vi "administrator.vi"(0 "vi path":path) -> ()   [LabVIEW 2010]
panel:
  in  "Test Number":string
  in  "User":string
  in  "OK Button":bool
  out "File path":string
  out "User Name 2":string caption="User Name"
  in  "Exit Modify":bool
  in  "Replace":bool
  in  "New Password":string
  in  "New Name":string
  in  "New Group":u16(ring) items=["admin", "user"]
  out "Username                  Tests Completed   Priviledges":string[][](array[string])
  in  "Exit":bool
  in  "Modify":bool
  out "Password":string
  out "Group":u16(ring) items=["admin", "user"]
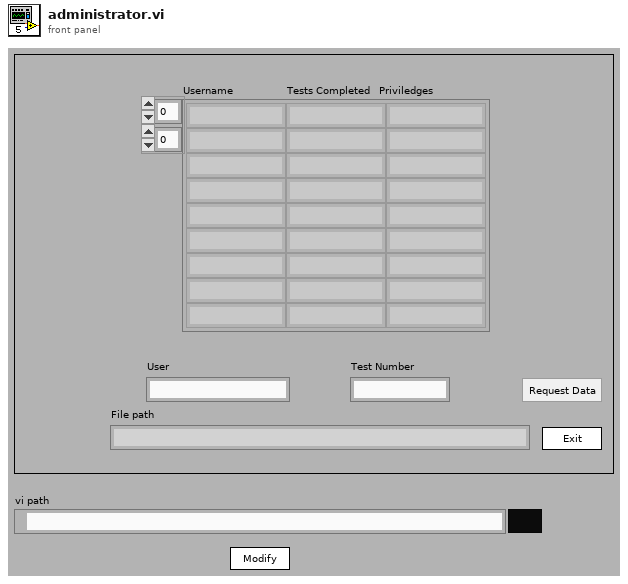
[diagram p1: front panel]
types:
  T1 = enum16{"open", "open or create", "create or replace", "create", "open (read only)"}
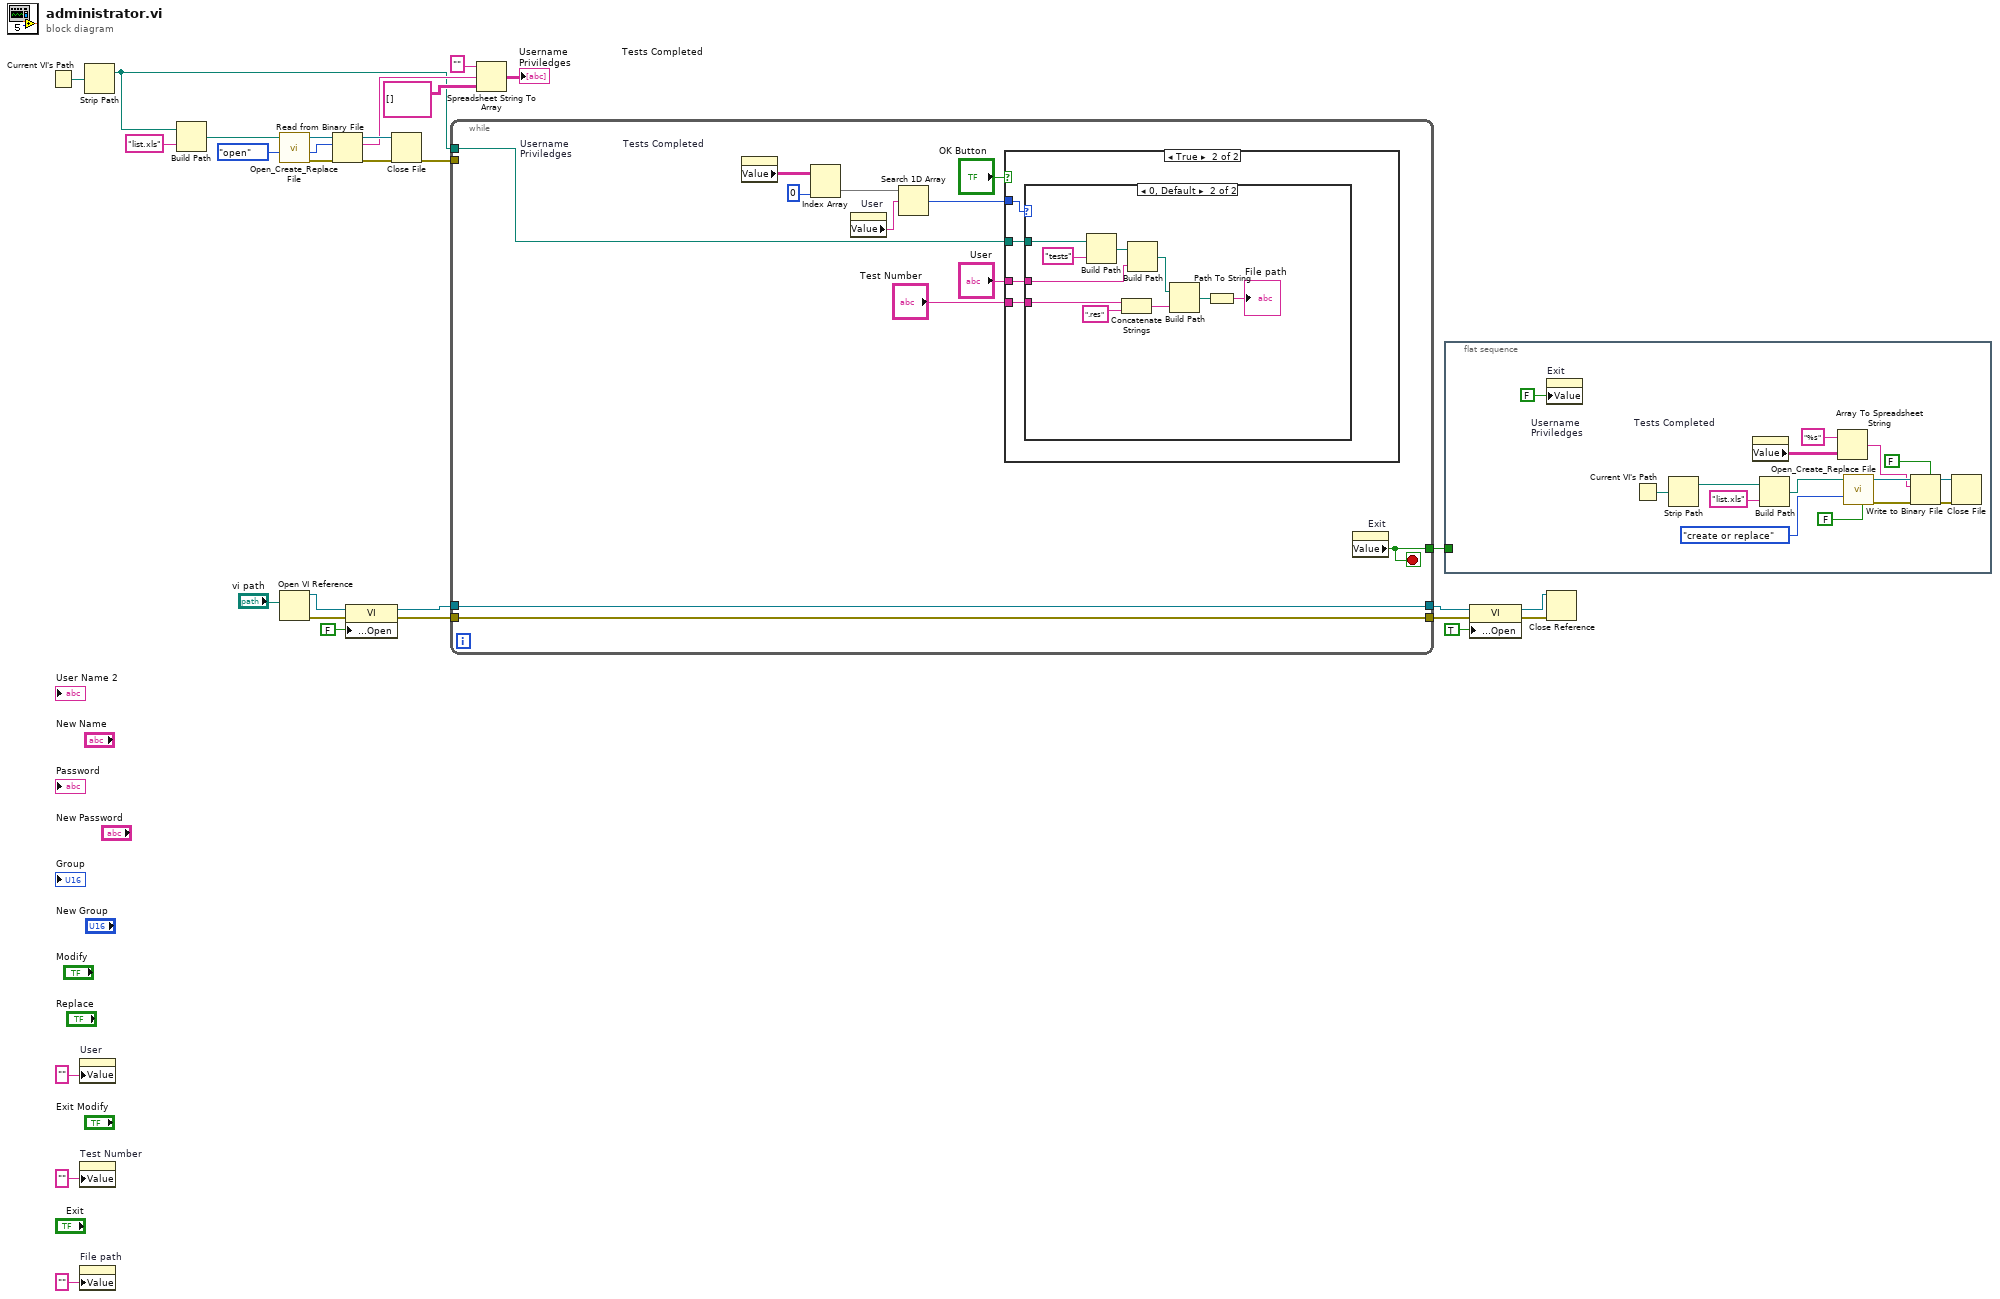
[diagram p0: block diagram]
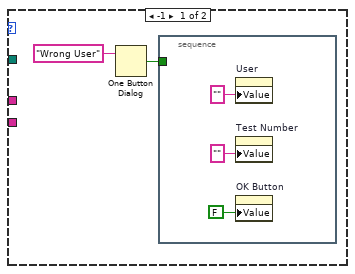
[diagram p3: hidden frame]
diagram:
  n1 = Current VI's Path() -> (path=w7:path)
  n2 = property on="User" class="Str"("Value"="" ("String")) -> ()  [unwired: 2 in, 2 out]
  n3 = property on="Test Number" class="Str"("Value"="" ("String")) -> ()  [unwired: 2 in, 2 out]
  n4 = property on="File path" class="Str"("Value"="" ("String")) -> ()  [unwired: 2 in, 2 out]
  n5 = Strip Path(path=w7) -> (stripped path=w1:path)  [unwired: 1 out]
  n6 = Build Path(base path=w1, name or relative path="list.xls") -> (appended path=w5:path)
  n7 = call <vilib>:"Open_Create_Replace File.vi"("function (open:0)"=T1."open", "file path"=w5) -> ("error out"=w30:errorcluster, "file size (bytes)"=w26:i32, "refnum"=w29:refnum<file>)  [unwired: 6 in, 1 out]
  n8 = Open VI Reference(vi path="vi path") -> (vi reference=w17:refnum<vi>, error out=w16:errorcluster)  [unwired: 5 in]
  n9 = Read from Binary File(8:w30, 10:w26, 11:w29) -> (0:w28:errorcluster, 2:w25:string, 3:w27:refnum<file>)  [unwired: 3 in, 1 out]
  n10 = property class="VI"(reference=w17, error in=w16, "Front Panel Window:Open"=FALSE) -> (reference out=w14:refnum<vi>, error out=w13:errorcluster)
  n11 = Close File(refnum=w27, error in=w28) -> (error out=w20:errorcluster)  [unwired: 1 out]
  n12 = while {
    tunnel: w20 -> [_]
    tunnel: [w42] -> w19
    tunnel: w14 -> [w41]
    tunnel: w13 -> [w40]
    tunnel: [w41] -> w11
    tunnel: [w40] -> w10
    tunnel: w1 -> [w39]
    stop <- w42 stop-if-true
    n13 = property on="Username                  Tests Completed   Priviledges" class="Arr (strict)"() -> ("Value"=w32:string[][])  [unwired: 2 in, 2 out]
    n14 = Index Array(array=w32, index (col)=0 ("disabled index (col)")) -> (element=w33:string[])  [unwired: 1 in]
    n15 = property on="User" class="Str"() -> ("Value"=w35:string)  [unwired: 2 in, 2 out]
    n16 = Search 1D Array(1D array=w33, element=w35) -> (index of element=w31:i32)  [unwired: 1 in]
    n17 = case shown="True" "OK Button" {
      tunnel: "User" -> [_ w46]
      tunnel: "Test Number" -> [_ w45]
      tunnel: w39 -> [_ w44]
      tunnel: w31 -> [_ w43]
      frame False {
      }
      frame True {
        n18 = case shown="0, Default" w43 {
          tunnel: w46 -> [_ w55]
          tunnel: w45 -> [_ w57]
          tunnel: w44 -> [_ w53]
          frame -1 {
            n19 = One Button Dialog(message="Wrong User") -> (true=w47:bool)  [unwired: 1 in]
            n20 = stacked-sequence {
              tunnel: w47 -> [_]
              frame #0 {
                n21 = property on="User" class="Str"("Value"="" ("Password")) -> ()  [unwired: 2 in, 2 out]
                n22 = property on="Test Number" class="Str"("Value"="" ("Password")) -> ()  [unwired: 2 in, 2 out]
                n23 = property on="OK Button" class="Bool"("Value"=FALSE ("true")) -> ()  [unwired: 2 in, 2 out]
              }
            }
          }
          frame 0, Default {
            n24 = Build Path(base path=w53, name or relative path="tests") -> (appended path=w54:path)
            n25 = Concatenate Strings(w57, ".res" ("string")) -> (w61:string)
            n26 = Build Path(base path=w54, name or relative path=w55) -> (appended path=w58:path)
            n27 = Build Path(base path=w58, name or relative path=w61) -> (appended path=w59:path)
            n28 = Path To String(path=w59) -> (string=→"File path":string)
          }
        }
      }
    }
    n29 = property on="Exit" class="Bool (strict)"() -> ("Value"=w42:bool)  [unwired: 2 in, 2 out]
  }
  n30 = Spreadsheet String To Array(format string="", spreadsheet string=w25, array type (2D Dbl)=string[][] []) -> (array=→"Username                  Tests Completed   Priviledges":string[][])  [unwired: 1 in]
  n31 = flat-sequence {
    tunnel: w19 -> [_]
    frame #0 {
      n32 = property on="Exit" class="Bool (strict)"("Value"=FALSE ("ADD")) -> ()  [unwired: 2 in, 2 out]
      n33 = Current VI's Path() -> (path=w66:path)
      n34 = Strip Path(path=w66) -> (stripped path=w65:path)  [unwired: 1 out]
      n35 = property on="Username                  Tests Completed   Priviledges" class="Arr (strict)"() -> ("Value"=w71:string[][])  [unwired: 2 in, 2 out]
      n36 = Build Path(base path=w65, name or relative path="list.xls") -> (appended path=w63:path)
      n37 = Array To Spreadsheet String(array=w71, 3:"%s" ("format string")) -> (spreadsheet string=w70:string)  [unwired: 1 in]
      n38 = call <vilib>:"Open_Create_Replace File.vi"("advisory dialog? (display:T)"=FALSE, "function (open:0)"=T1."create or replace", "file path"=w63) -> ("error out"=w72:errorcluster, "refnum"=w73:refnum<file>)  [unwired: 5 in, 2 out]
      n39 = Write to Binary File(file (use dialog)=w73, data=w70, error in=w72, 5:FALSE ("prepend array or string size? (T)")) -> (refnum out=w75:refnum<file>, error out=w74:errorcluster)  [unwired: 2 in, 1 out]
      n40 = Close File(refnum=w75, error in=w74) -> ()  [unwired: 2 out]
    }
  }
  n41 = property class="VI"(reference=w11, error in=w10, "Front Panel Window:Open"=TRUE) -> (reference out=w9:refnum<vi>, error out=w8:errorcluster)
  n42 = Close Reference(reference=w9, error in (no error)=w8) -> ()  [unwired: 1 out]
